vi "log.vi"(0 "worker":i8, 2 "input string":string) -> (5 "all workers_log":string[](array[string]), 6 "worker_log":string[](array[string]), 8 "current log":string)   [LabVIEW 2023]
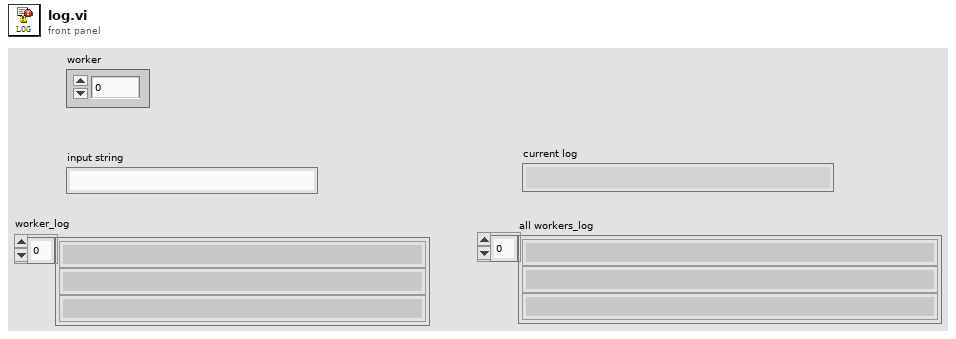
[diagram p1: front panel]
types:
  T1 = enum16{"open", "replace", "create", "open or create", "replace or create", "replace or create with confirmation"}
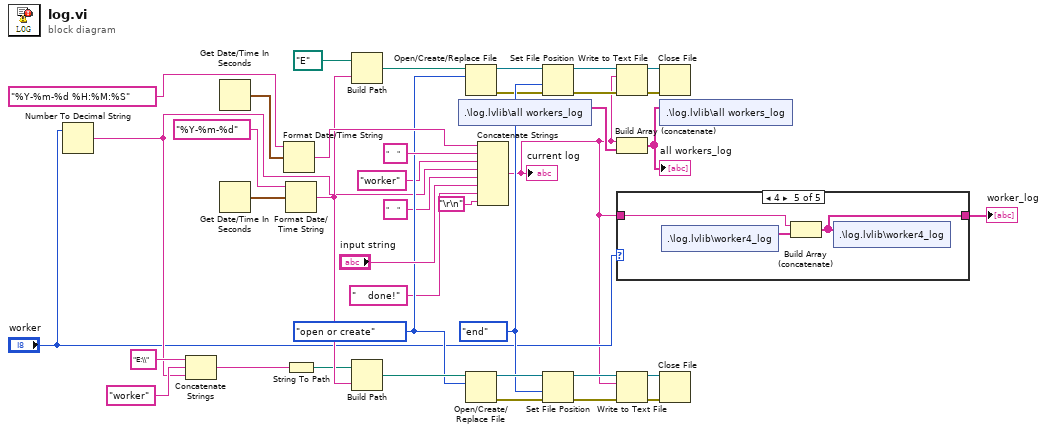
[diagram p0: block diagram]
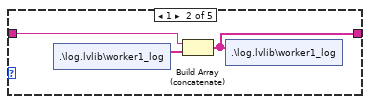
[diagram p3: hidden frame]
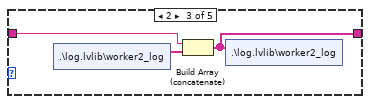
[diagram p4: hidden frame]
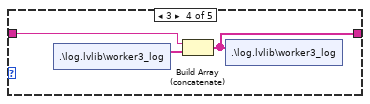
[diagram p5: hidden frame]
diagram:
  w20 = enum16{"start", "end", "current"}."end" ("from (0:start)")
  w21 = T1."open or create" ("operation (0:open)")
  n1 = Number To Decimal String(number="worker") -> (decimal integer string=w6:string)  [unwired: 1 in]
  n2 = Concatenate Strings("E:\\" ("time format string (%c)"), "worker" ("time format string (%c)"), w6) -> (w12:string)
  n3 = Get Date/Time In Seconds() -> (seconds since 1Jan1904=w38:timestamp)
  n4 = Get Date/Time In Seconds() -> (seconds since 1Jan1904=w26:timestamp)
  n5 = Format Date/Time String(time format string (%c)="%Y-%m-%d %H:%M:%S", seconds (now)=w38) -> (date/time string=w34:string)  [unwired: 1 in]
  n6 = Format Date/Time String(time format string (%c)="%Y-%m-%d", seconds (now)=w26) -> (date/time string=w23:string)  [unwired: 1 in]
  n7 = String To Path(string=w12) -> (path=w9:path)
  n8 = Build Path(base path=path "E:/", name or relative path=w23) -> (appended path=w22:path)
  n9 = Build Path(base path=w9, name or relative path=w23) -> (appended path=w37:path)
  n10 = shared-variable ".\\log.lvlib\\all workers_log"() -> (w2:string[])  [unwired: 1 in, 1 out]
  n11 = Open/Create/Replace File(file path (use dialog)=w22, operation (0:open)=w21) -> (refnum out=w19:refnum<file>, error out=w18:errorcluster)  [unwired: 4 in, 1 out]
  n12 = Open/Create/Replace File(file path (use dialog)=w37, operation (0:open)=w21) -> (refnum out=w33:refnum<file>, error out=w32:errorcluster)  [unwired: 4 in, 1 out]
  n13 = Concatenate Strings(w34, "    " ("string"), "worker" ("time format string (%c)"), w6, "    " ("string"), "input string", "    done!" ("string"), "\r\n") -> (w1:string)
  "current log" <- w1
  n14 = Set File Position(refnum=w19, from (0:start)=w20, error in=w18) -> (refnum out=w17:refnum<file>, error out=w16:errorcluster)  [unwired: 1 in]
  n15 = Set File Position(refnum=w33, from (0:start)=w20, error in=w32) -> (refnum out=w31:refnum<file>, error out=w30:errorcluster)  [unwired: 1 in]
  n16 = Write to Text File(file (use dialog)=w17, text=w1, error in=w16) -> (refnum out=w13:refnum<file>, error out=w14:errorcluster)  [unwired: 1 in, 1 out]
  n17 = Build Array (concatenate)(w1, w2) -> (w15:string[])
  "all workers_log" <- w15
  n18 = case shown="4" "worker" {
    tunnel: w1 -> [_ w40 w44 w47 w50]
    tunnel: [_ w42 w45 w48 w51] -> w3
    frame 0, Default {
    }
    frame 1 {
      n19 = shared-variable ".\\log.lvlib\\worker1_log"() -> (w41:string[])  [unwired: 1 in, 1 out]
      n20 = Build Array (concatenate)(w40, w41) -> (w42:string[])
      n21 = shared-variable ".\\log.lvlib\\worker1_log"(w42) -> ()  [unwired: 1 in, 1 out]
    }
    frame 2 {
      n22 = shared-variable ".\\log.lvlib\\worker2_log"() -> (w43:string[])  [unwired: 1 in, 1 out]
      n23 = Build Array (concatenate)(w44, w43) -> (w45:string[])
      n24 = shared-variable ".\\log.lvlib\\worker2_log"(w45) -> ()  [unwired: 1 in, 1 out]
    }
    frame 3 {
      n25 = shared-variable ".\\log.lvlib\\worker3_log"() -> (w46:string[])  [unwired: 1 in, 1 out]
      n26 = Build Array (concatenate)(w47, w46) -> (w48:string[])
      n27 = shared-variable ".\\log.lvlib\\worker3_log"(w48) -> ()  [unwired: 1 in, 1 out]
    }
    frame 4 {
      n28 = shared-variable ".\\log.lvlib\\worker4_log"() -> (w49:string[])  [unwired: 1 in, 1 out]
      n29 = Build Array (concatenate)(w50, w49) -> (w51:string[])
      n30 = shared-variable ".\\log.lvlib\\worker4_log"(w51) -> ()  [unwired: 1 in, 1 out]
    }
  }
  "worker_log" <- w3
  n31 = Write to Text File(file (use dialog)=w31, text=w1, error in=w30) -> (refnum out=w35:refnum<file>, error out=w36:errorcluster)  [unwired: 1 in, 1 out]
  n32 = Close File(refnum=w13, error in=w14) -> ()  [unwired: 2 out]
  n33 = shared-variable ".\\log.lvlib\\all workers_log"(w15) -> ()  [unwired: 1 in, 1 out]
  n34 = Close File(refnum=w35, error in=w36) -> ()  [unwired: 2 out]
